vi "PWC Cluster.vi"(2 "Return Indicies":bool, 3 "Kernel Precission Parameter":dbl, 4 "# Cluster Levels":i32, 5 "Input Waveform":dbl[](array[numeric])) -> (0 "Converged":bool, 1 "Cluster Assignments":dbl[](array[numeric]))   [LabVIEW 2013]
uses:
  <vilib>/Analysis/baseanly.llb/A x Vector.vi
  <vilib>/Analysis/Matrix/Numeric/Conversions/Array To Matrix - RA2.vi
  <vilib>/Analysis/Matrix/NI_Matrix.lvlib
  <vilib>/Analysis/NI_AALBase.lvlib
panel:
  out "Waveform Graph":dbl[][](graph)
  out "Cluster Centroids":dbl[](array[numeric])
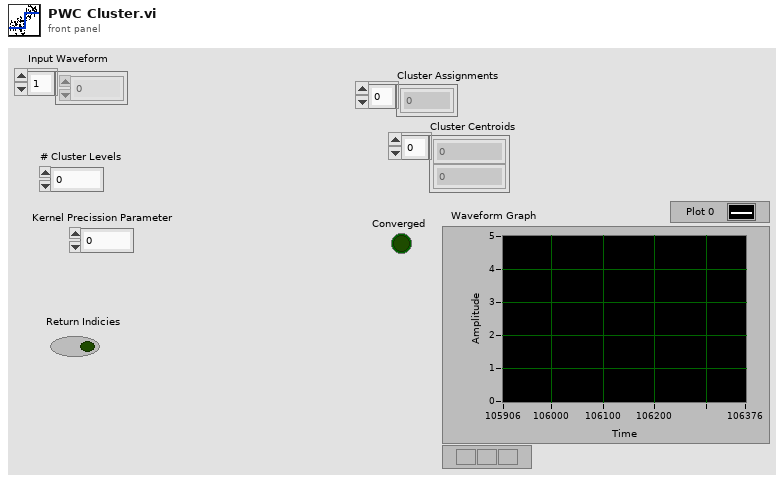
[diagram p1: front panel]
types:
  T1 = typedef "NI_Matrix.lvlib/RealMatrix.ctl" = dbl[][]
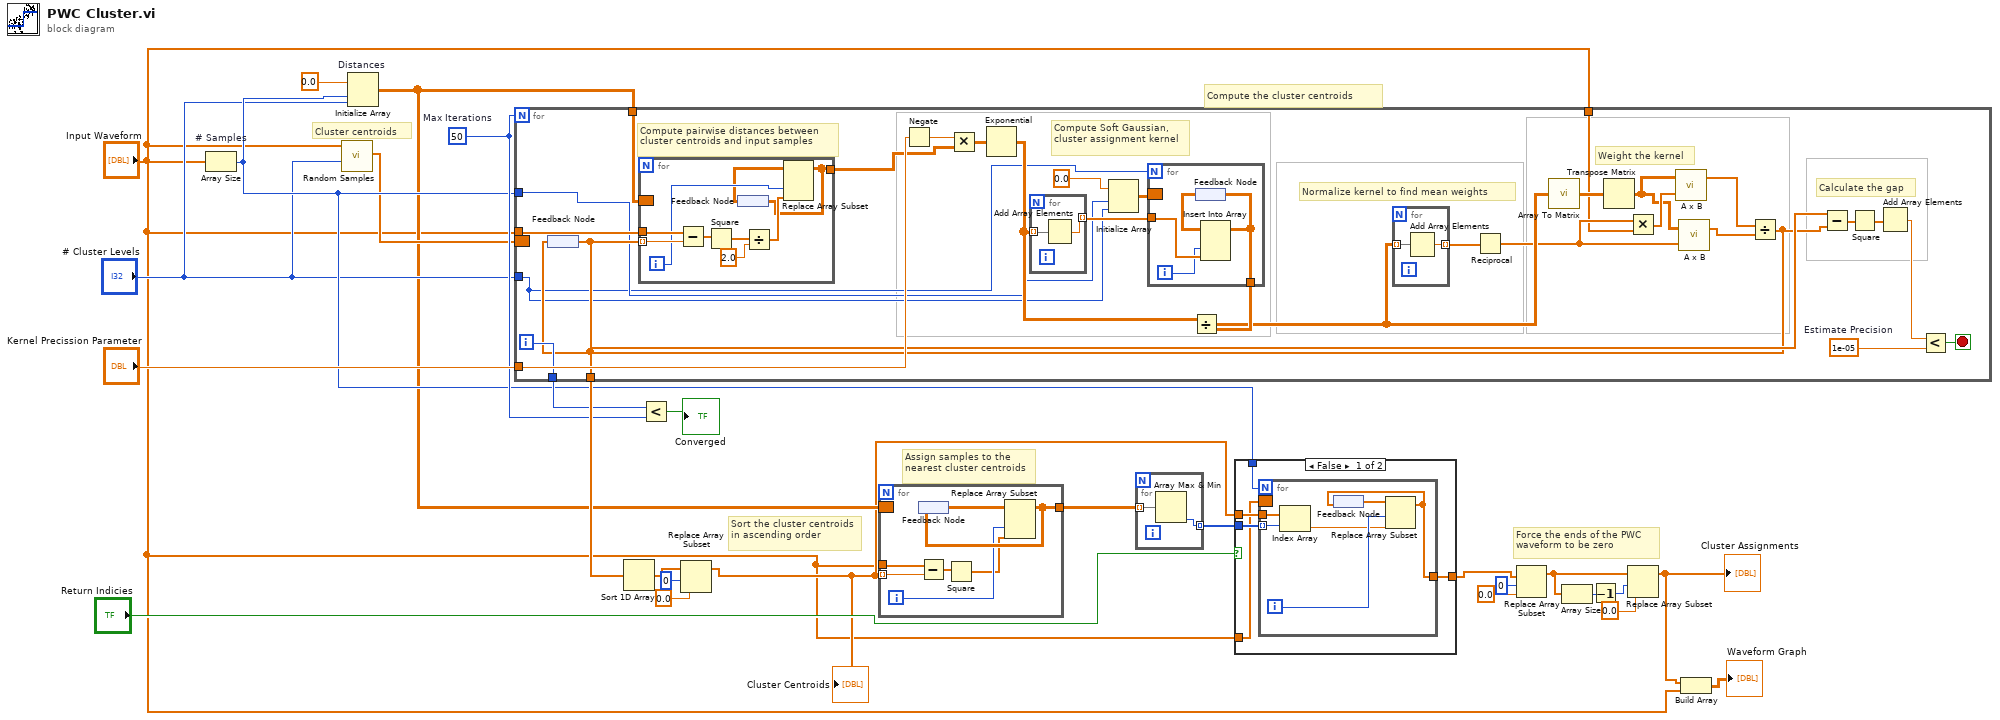
[diagram p0: block diagram]
diagram:
  w23 = 50  # Max Iterations
  # "Force the ends of the PWC waveform to be zero"
  # "Sort the cluster centroids in ascending order"
  # "Compute the cluster centroids"
  # "Assign samples to the nearest cluster centroids"
  # "Cluster centroids"
  n1 = Array Size "# Samples"(array="Input Waveform") -> (size(s)=w19:i32)
  n2 = call "Random Samples.vi"("# Picks"="# Cluster Levels", "Input Array"="Input Waveform") -> ("Samples"=w9:dbl[])  [unwired: 9 in]
  n3 = Initialize Array "Distances"(0.0 ("Constant"), w19, "# Cluster Levels") -> (w8:dbl[][])
  n4 = for {
    N: w23 -> [_]
    tunnel: "# Cluster Levels" -> [w29]
    tunnel: w8 -> [w32]
    tunnel: "Input Waveform" -> [w54]
    tunnel: "Kernel Precission Parameter" -> [w47]
    tunnel: "Input Waveform" -> [w39]
    tunnel: [w34] -> w25
    tunnel: w19 -> [w30]
    tunnel: [w35] -> w24
    border: w9 -> [_]
    i -> [w35]
    stop <- w57 stop-if-true
    w41 = 1e-05  # Estimate Precision
    # "Compute Soft Gaussian, cluster assignment kernel"
    # "Compute pairwise distances between\ncluster centroids and input samples"
    # "Calculate the gap"
    # "Weight the kernel"
    # "Normalize kernel to find mean weights"
    n5 = feedback #1() -> (w38:dbl[])
    n6 = for {
      tunnel: w54 -> [w72]
      tunnel: w38 -> [w71] mode=indexing
      tunnel: [w64] -> w33
      border: w32 -> [_]
      i -> [w67]
      n7 = Subtract(x=w72, y=w71) -> (x-y=w70:dbl[])
      n8 = Square(x=w70) -> (x^2=w69:dbl[])
      n9 = feedback #2() -> (w65:dbl[][])
      n10 = Divide(x=w69, y=2.0 ("value")) -> (x/y=w66:dbl[])
      n11 = Replace Array Subset(array=w65, new element=w66, index (col)=w67) -> (w64:dbl[][])  [unwired: 1 in]
      n12 = feedback-in #2(w64) -> ()
    }
    n13 = Negate(x=w47) -> (-x=w53:dbl)
    n14 = Multiply(x=w53, y=w33) -> (x*y=w52:dbl[][])
    n15 = Exponential(1:w52) -> (0:w49:dbl[][])
    n16 = for {
      tunnel: w49 -> [w63] mode=indexing
      tunnel: [w62] -> w51 mode=indexing
      n17 = Add Array Elements(numeric array=w63) -> (sum=w62:dbl)
    }
    n18 = Initialize Array(0.0 ("element"), w30, w29) -> (w28:dbl[][])
    n19 = for {
      N: w29 -> [_]
      tunnel: w51 -> [w61]
      tunnel: [w58] -> w50
      border: w28 -> [_]
      i -> [w59]
      n20 = feedback #3() -> (w60:dbl[][])
      n21 = Insert Into Array(array=w60, index (col)=w59, new element=w61) -> (w58:dbl[][])  [unwired: 1 in]
      n22 = feedback-in #3(w58) -> ()
    }
    n23 = Divide(x=w49, y=w50) -> (x/y=w48:dbl[][])
    n24 = for {
      tunnel: w48 -> [w74] mode=indexing
      tunnel: [w73] -> w56 mode=indexing
      n25 = Add Array Elements(numeric array=w74) -> (sum=w73:dbl)
    }
    n26 = Reciprocal(x=w56) -> (1/x=w40:dbl[])
    n27 = call-poly <vilib>:"Array To Matrix.vi"("Real 2D Array"=w48) -> ("Real Matrix"=w42:T1)
    n28 = Transpose Matrix(1:w42) -> (0:w45:T1)
    n29 = Multiply ("Multiply.vi")(x=w40, y=w39) -> (x*y=w46:dbl[])
    n30 = call-poly <vilib>:"A x B.vi"("Vector"=w46, "A"=w45) -> ("A x Vector"=w44:dbl[])  [unwired: 1 out]
    n31 = call-poly <vilib>:"A x B.vi"("Vector"=w40, "A"=w45) -> ("A x Vector"=w43:dbl[])  [unwired: 1 out]
    n32 = Divide(x=w44, y=w43) -> (x/y=w34:dbl[])
    n33 = feedback-in #1(w34) -> ()
    n34 = Subtract ("Subtract.vi")(x=w38, y=w34) -> (x-y=w55:dbl[])
    n35 = Square(x=w55) -> (x^2=w37:dbl[])
    n36 = Add Array Elements(numeric array=w37) -> (sum=w36:dbl)
    n37 = Less?(x=w36, y=w41) -> (x < y?=w57:bool)
  }
  n38 = Sort 1D Array(array=w25) -> (sorted array=w7:dbl[])
  n39 = Less?(x=w24, y=w23) -> (x < y?=→"Converged":bool)
  n40 = Replace Array Subset(array=w7, new element=0.0 ("new element/subarray"), index=0) -> (w4:dbl[])
  "Cluster Centroids" <- w4
  n41 = for {
    tunnel: [w79] -> w17
    tunnel: w4 -> [w77] mode=indexing
    tunnel: "Input Waveform" -> [w76]
    border: w8 -> [_]
    i -> [w78]
    n42 = feedback #4() -> (w80:dbl[][])
    n43 = Subtract(x=w76, y=w77) -> (x-y=w81:dbl[])
    n44 = Square(x=w81) -> (x^2=w75:dbl[])
    n45 = Replace Array Subset(array=w80, new element=w75, index (col)=w78) -> (w79:dbl[][])  [unwired: 1 in]
    n46 = feedback-in #4(w79) -> ()
  }
  n47 = for {
    tunnel: [w83] -> w20 mode=indexing
    tunnel: w17 -> [w82] mode=indexing
    n48 = Array Max & Min(array=w82) -> (min index (indices)=w83:i32)  [unwired: 3 out]
  }
  n49 = case shown="False" "Return Indicies" {
    tunnel: [w85 w95] -> w16
    tunnel: w20 -> [w87 w95]
    tunnel: w19 -> [w88 _]
    tunnel: "Input Waveform" -> [w84 _]
    tunnel: w4 -> [w86 _]
    frame False {
      n50 = for {
        N: w88 -> [_]
        tunnel: w87 -> [w91] mode=indexing
        tunnel: w86 -> [w92]
        tunnel: [w89] -> w85
        border: w84 -> [_]
        i -> [w93]
        n51 = Index Array(array=w92, index=w91) -> (element=w90:dbl)
        n52 = feedback #5() -> (w94:dbl[])
        n53 = Replace Array Subset(array=w94, new element=w90, index=w93) -> (w89:dbl[])
        n54 = feedback-in #5(w89) -> ()
      }
    }
    frame True {
      # "Return just the index of the cluster centroid that each sample belongs to"
    }
  }
  n55 = Replace Array Subset(array=w16, new element=0.0 ("new element/subarray"), index=0) -> (w13:dbl[])
  n56 = Array Size(array=w13) -> (size(s)=w10:i32)
  n57 = Decrement(x=w10) -> (x-1=w12:i32)
  n58 = Replace Array Subset(array=w13, new element=0.0 ("new element/subarray"), index=w12) -> (w3:dbl[])
  "Cluster Assignments" <- w3
  n59 = Build Array(w3, "Input Waveform") -> (→"Waveform Graph":dbl[][])
